vi "DSF.Engine.Execution.Builder.Get RT Thread Parameters.vi"(8 "error in (no error)":errorcluster, 11 "Builder in":refnum<class "DSF.Engine.Execution.Builder.lvclass">) -> (0 "error out":errorcluster, 2 "RT Thread Parameters":T1={"Priority"=100, "Processor"=-2}, 3 "Builder out":refnum<class "DSF.Engine.Execution.Builder.lvclass">)   [LabVIEW 2016, in "DSF.Engine.lvlib" / "DSF.Engine.Execution.Builder.lvclass"]
uses:
  Builder/DSF.Engine.Execution.Builder.lvclass
  Typedefs/DSF.Shared.RT Thread Parameters.ctl
  Builder/DSF.Engine.Execution.Builder.lvclass/DSF.Engine.Execution.Builder.ctl
  DSF.Shared.lvlib
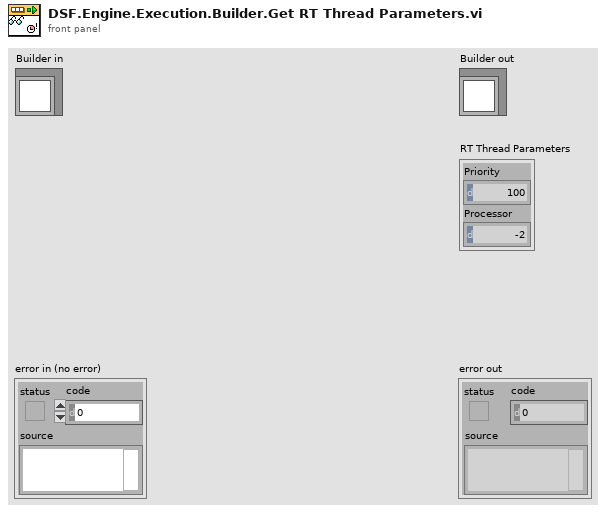
[diagram p1: front panel]
types:
  T1 = typedef "DSF.Shared.lvlib/DSF.Shared.RT Thread Parameters.ctl" = cluster{"Priority":i32, "Processor":i32}
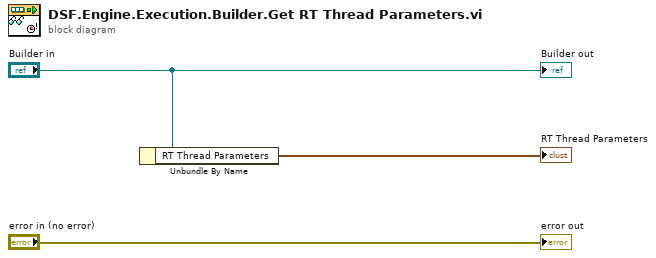
[diagram p0: block diagram]
diagram:
  n1 = Unbundle By Name("Builder in") -> ("RT Thread Parameters"=→"RT Thread Parameters":T1)
  "error out" <- "error in (no error)"
  "Builder out" <- "Builder in"
